vi "启动画面.vi"() -> ()   [LabVIEW 2018]
panel:
  out "进度条":u8(slide) scale=0.0..100.0
  # "该启动画面程序会显示子 VI 加载进度，然后调用主程序，\n最后关闭该启动画面，注意确保主程序当前没有运行"
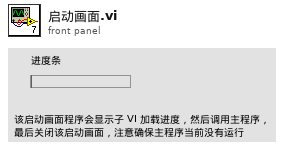
[diagram p1: front panel]
types:
  T1 = enum32{"Invalid", "Standard", "Closed", "Hidden", "Minimized", "Maximized"}
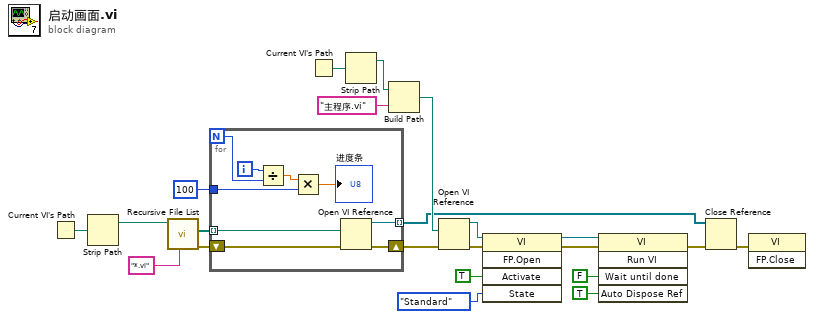
[diagram p0: block diagram]
diagram:
  n1 = Current VI's Path() -> (path=w22:path)
  n2 = Strip Path(path=w22) -> (stripped path=w18:path)  [unwired: 1 out]
  n3 = call <vilib>:"Recursive File List.vi"("pattern"="*.vi", "Folder Path"=w18) -> ("error out"=w19:errorcluster, "All Files in Dir"=w20:path[])  [unwired: 5 in, 3 out]
  n4 = for {
    N -> [w28]
    tunnel: w20 -> [w31] mode=indexing
    shift-right: [w29] -> w14
    shift-left: w19 -> [w30]
    tunnel: [w26] -> w7 mode=indexing
    tunnel: 100 -> [w24]
    i -> [w27]
    n5 = Divide(x=w27, y=w28) -> (x/y=w25:dbl)
    n6 = Multiply(x=w25, y=w24) -> (x*y=→"进度条":dbl)
    n7 = Open VI Reference(vi path=w31, error in (no error)=w30) -> (vi reference=w26:refnum<vi>, error out=w29:errorcluster)  [unwired: 4 in]
  }
  n8 = Current VI's Path() -> (path=w13:path)
  n9 = Strip Path(path=w13) -> (stripped path=w12:path)  [unwired: 1 out]
  n10 = Build Path(base path=w12, name or relative path="主程序.vi" ("名称或相对路径")) -> (appended path=w17:path)
  n11 = Open VI Reference(vi path=w17, error in (no error)=w14) -> (vi reference=w15:refnum<vi>, error out=w11:errorcluster)  [unwired: 4 in]
  n12 = invoke class="VI" method="FP.Open"(reference=w15, error in=w11, "Activate"=TRUE ("激活？"), "State"=T1."Standard" ("状态")) -> (reference out=w9:refnum<vi>, error out=w1:errorcluster)  [unwired: 1 in, 3 out]
  n13 = invoke class="VI" method="Run VI"(reference=w9, error in=w1, "Wait until done"=FALSE ("结束前等待"), "Auto Dispose Ref"=TRUE ("自动销毁引用")) -> (error out=w8:errorcluster)  [unwired: 1 in, 4 out]
  n14 = Close Reference(reference=w7, error in (no error)=w8) -> (error out=w6:errorcluster)
  n15 = invoke class="VI" method="FP.Close"(error in=w6) -> ()  [unwired: 2 in, 3 out]
